vi "clone.vi"(0 "reference":refnum<class "InitialStateNode.lvclass">, 5 "error in (no error)":errorcluster) -> (14 "reference out":refnum<class "InitialStateNode.lvclass">, 15 "clonedInterfaceNode":refnum<class "AbstractNode.lvclass">, 19 "error out":errorcluster)   [LabVIEW 2020, in "InitialStateNode.lvclass"]
doc: "public Object clone()"
uses:
  <resource>/Framework/Providers/Open_GDS/UML/InitialStateNode_class/InitialStateNode.lvclass
  C:/Program Files (x86)/National Instruments/LabVIEW 2020/resource/Framework/Providers/Open_GDS/UML/RectangularNode_class/RectangularNode.lvclass
  C:/Program Files (x86)/National Instruments/LabVIEW 2020/resource/Framework/Providers/Open_GDS/UML/AbstractNode_class/AbstractNode.lvclass
  <resource>/Framework/Providers/Open_GDS/UML/AbstractNode_class/AbstractNode.lvclass
  <resource>/Framework/Providers/Open_GDS/UML/MultiLineString_class/MultiLineString.lvclass
  <resource>/Framework/Providers/Open_GDS/UML/RectangularNode_class/RectangularNode.lvclass
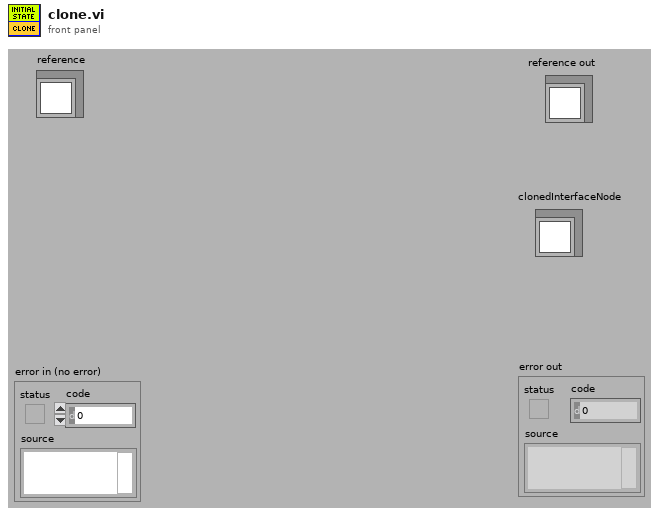
[diagram p1: front panel]
types:
  T1 = typedef "RectangularNode.lvclass/ObjectAttributes.ctl" = cluster{"bounds":T2}
  T2 = typedef "Rectangle Rectangle2D.ctl" = cluster{"x":dbl, "y":dbl, "width":dbl, "height":dbl}
  T3 = typedef "InitialStateNode.lvclass/ObjectAttributes.ctl" = cluster{"name":refnum<class "MultiLineString.lvclass">, "DEFAULT_WIDTH":i32, "DEFAULT_HEIGHT":i32}
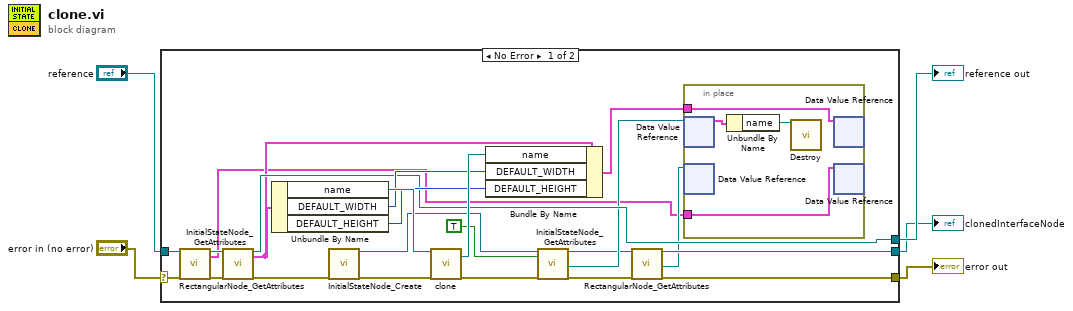
[diagram p0: block diagram]
diagram:
  n1 = case shown="No Error" "error in (no error)" {
    selector: "error in (no error)" -> [w28 w33]
    tunnel: "reference" -> [w12 w34]
    tunnel: [w10 w33] -> w4
    tunnel: [w19 w34] -> w3
    tunnel: [w8 _] -> w1
    frame No Error {
      n2 = call <resource>:"RectangularNode_GetAttributes.vi"("reference in"=w12, "error in (no error)"=w28) -> ("reference out"=w11:refnum<class "InitialStateNode.lvclass">, "Data"=w6:T1, "error out"=w13:errorcluster)  [unwired: 14 in, 1 out]
      n3 = call <resource>:"InitialStateNode_GetAttributes.vi"("reference in"=w11, "error in (no error)"=w13) -> ("reference out"=w19:refnum<class "InitialStateNode.lvclass">, "Data"=w17:T3, "error out"=w20:errorcluster)  [unwired: 1 in, 14 out]
      n4 = Unbundle By Name(w17) -> ("name"=w26:refnum<class "MultiLineString.lvclass">, "DEFAULT_WIDTH"=w22:i32, "DEFAULT_HEIGHT"=w21:i32)
      n5 = call <resource>:"InitialStateNode_Create.vi"("error in (no error)"=w20) -> ("reference out"=w23:refnum<class "InitialStateNode.lvclass">, "error out"=w27:errorcluster)  [unwired: 17 in]
      n6 = call-dynamic "clone.vi"("reference"=w26, "error in (no error)"=w27) -> ("clonedMultiLineString"=w25:refnum<class "MultiLineString.lvclass">, "error out"=w24:errorcluster)  [unwired: 15 in, 1 out]
      n7 = Bundle By Name(cluster=w17, "name"=w25, "DEFAULT_WIDTH"=w22, "DEFAULT_HEIGHT"=w21) -> (w14:T3)
      n8 = call <resource>:"InitialStateNode_GetAttributes.vi"("reference in"=w23, "OnlyGetDvrReference(False)"=TRUE, "error in (no error)"=w24) -> ("reference out"=w9:refnum<class "InitialStateNode.lvclass">, "DataRef"=w15:refnum<data-value>, "error out"=w16:errorcluster)  [unwired: 13 in, 1 out]
      n9 = call <resource>:"RectangularNode_GetAttributes.vi"("reference in"=w9, "error in (no error)"=w16) -> ("reference out"=w8:refnum<class "InitialStateNode.lvclass">, "DataRef"=w7:refnum<data-value>, "error out"=w10:errorcluster)  [unwired: 14 in, 1 out]
      n10 = in-place {
        in-place-border: w14 -> [w32]
        in-place-border: w6 -> [w29]
        n11 = in-place-dvr #1(w15) -> (w30:T3)  [unwired: 1 out]
        n12 = in-place-dvr #2(w7) -> ()  [unwired: 2 out]
        n13 = Unbundle By Name(w30) -> ("name"=w31:refnum<class "MultiLineString.lvclass">)
        n14 = call-dynamic "Destroy.vi"("reference"=w31) -> ()  [unwired: 17 in, 2 out]
        n15 = in-place-dvr #1(w32) -> ()  [unwired: 2 out]
        n16 = in-place-dvr #2(w29) -> ()  [unwired: 2 out]
      }
    }
    frame Error {
    }
  }
  "reference out" <- w3
  "error out" <- w4
  "clonedInterfaceNode" <- w1
